vi "ExAdvPMAppCamera.vi"() -> ()   [LabVIEW 2010]
uses:
  Open-Close/CamHandle.vi
  GlobalCCDMaxDim.vi
  GlobalInitializeFlag.vi
  GlobalFramesToStr.vi
  GlobalTimingMode.vi
  GlobalAcquireFocusFlag.vi
  GlobalExposure.vi
  GlobalUserBin.vi
  GlobalBin2x.vi
  GlobalFullBin.vi
  GlobalFlipFlag.vi
  GlobalReverseFlag.vi
  GlobalIBackImgHndl.vi
  GlobalIFlatImgHndl.vi
panel:
  out "Camera Opened 2":bool
  out "Camera Opened":bool
  in  "Exit program":bool
  out "error out":errorcluster
  in  "error in (no error)":errorcluster
  in  "Tab Control":T1(tab)
  in  "Focus/Acquire Mode":u32=1 min=1 max=5 step=1
  in  "Number of Frames to store":u32=1 min=1 step=1
  in  "Intensifier":bool
  in  "Readout Port":i32=-1 min=-1 step=1
  in  "ADC Offset 2":i32=-1 min=-1 step=1
  in  "ADC Gain 2":i32=-1 min=-1 step=1
  in  "ADC speed":i32=-2 min=-3 step=1
  in  "Trigger Edge":u32(ring)=1 items=["N/A", "Positive (leading) edge", "Negative (falling) edge"]
  in  "Timing Mode":u32(ring)=1 items=["N/A", "Free Run/Timed", "Trigger First (PM only)", "Ext Sync/Strobed ", "Variable Exp (PM only)", "Flash Mode (PM only)"]
  out "Pixel Time":i32
  out "Bit Depth":i32
  out "ReadOut port":i32
  out "ADC Offset":i32
  out "ADC Gain":i32
  out "ADC Speed":i32
  in  "Set Experiment \nParameters, Initialize \nCamera/Controller":bool
  out "temperature":dbl format="%.2f"
  out "Temperature Read":dbl(slide) scale=-120.0..20.0
  in  "Temperature":dbl format="%.2f"
  in  "Exposure":dbl format="%.2f"
  out "Controller Initialized":bool
  out "Total":u32
  out "Y dim":u32
  out "X dim":u32
  in  "Y Bin":u32=1 min=1 step=1
  in  "Y End":u32=100 min=1 step=1
  in  "Y Start":u32=1 min=1 step=1
  in  "X Bin":u32=1 min=1 step=1
  in  "X End":u32=100 min=1 step=1
  in  "X Start":u32=1 min=1 step=1
  out "Bin 2":bool
  out "User":bool
  out "Full":bool
  in  "Binned by 2 Button":bool
  in  "User Defined Button":bool
  in  "Full CCD Button":bool
  out "Flip\nActive":bool
  in  "Flip flag Button":bool
  out "Reverse\nActive":bool
  in  "Image Reverse Button":bool
  out "Flat Field\nActive":bool
  out "Background \nActive":bool
  in  "Frame number to read":u32=1 min=1 step=1
  in  "Flat Button":bool
  in  "Back Button":bool
  in  "Full File Name":path
  in  "FileType":u32=67371008
  in  "SITKFULLDISPLAYLib.SITKFullDisplay":refnum<k7>(container)
  out "Reverse\nactive":bool
  out "Flip\nactive":bool
  out "Flat Field\nactive":bool
  out "background\nactive":bool
  in  "Reverse\nbutton":bool
  in  "Flip\nbutton":bool
  in  "Flat Field\nbutton":bool
  in  "Background\nbutton":bool
  in  "stop 2":bool
  in  "Start":bool
  out "Camera initialized":bool
  out "Collecting Data":bool
  in  "SITKFULLDISPLAYLib.SITKFullDisplay":refnum<k7>(container)
  in  "Full File Name\nfor Acqure":path
  in  "OK Button":bool
  out "camera initialized":bool
  # "Note: In order for any parameters to change and be downloaded the initialize button must be hit."
  # "The following are read \nfrom camera after setting\nvalues to left.\n-1 value means it isn't \nsupported by camera."
  # "For Slowest ADC speed set this to -3\nFor Fastest ADC speed set this to -2\nTo use current ADC speed don't  hook up or use -1\notherwise put speed in as kHz"
  # "To use current gain don't hook up or set to -1"
  # "To use current gain don't hook up or set to -1"
  # "To use current gain don't hook up or set to -1"
  # "Pixels coming back\nfrom Camera"
  # "NOTE: if background subtraction and/or flat field are being used and \nthe ROIs changed, there are no checks in this example for this."
  # "File Types:\nSPE = 67371008\nTIF   = 67174400\nPMI  = 67436544"
  # "Browse match pattern is set to *.spe.  Modify this if different file type is needed."
  # "Instructions:\nMake sure camera/controller has been initialized (LED should be on).\nPress start button, display should appear.\nWhen done press stop button, display should disappear.\nLive Operations buttons only work while collecting data, not before,\nto setup before goto On-Line operations tab."
  # "Live Operations, will only work while collecting data."
  # "Instructions:\nMake sure the camera/controller has been initialized.  The light should be on.\nMake sure to put in a file name with path to save data.\nPress Start button and display will pop up and data will be saved in file."
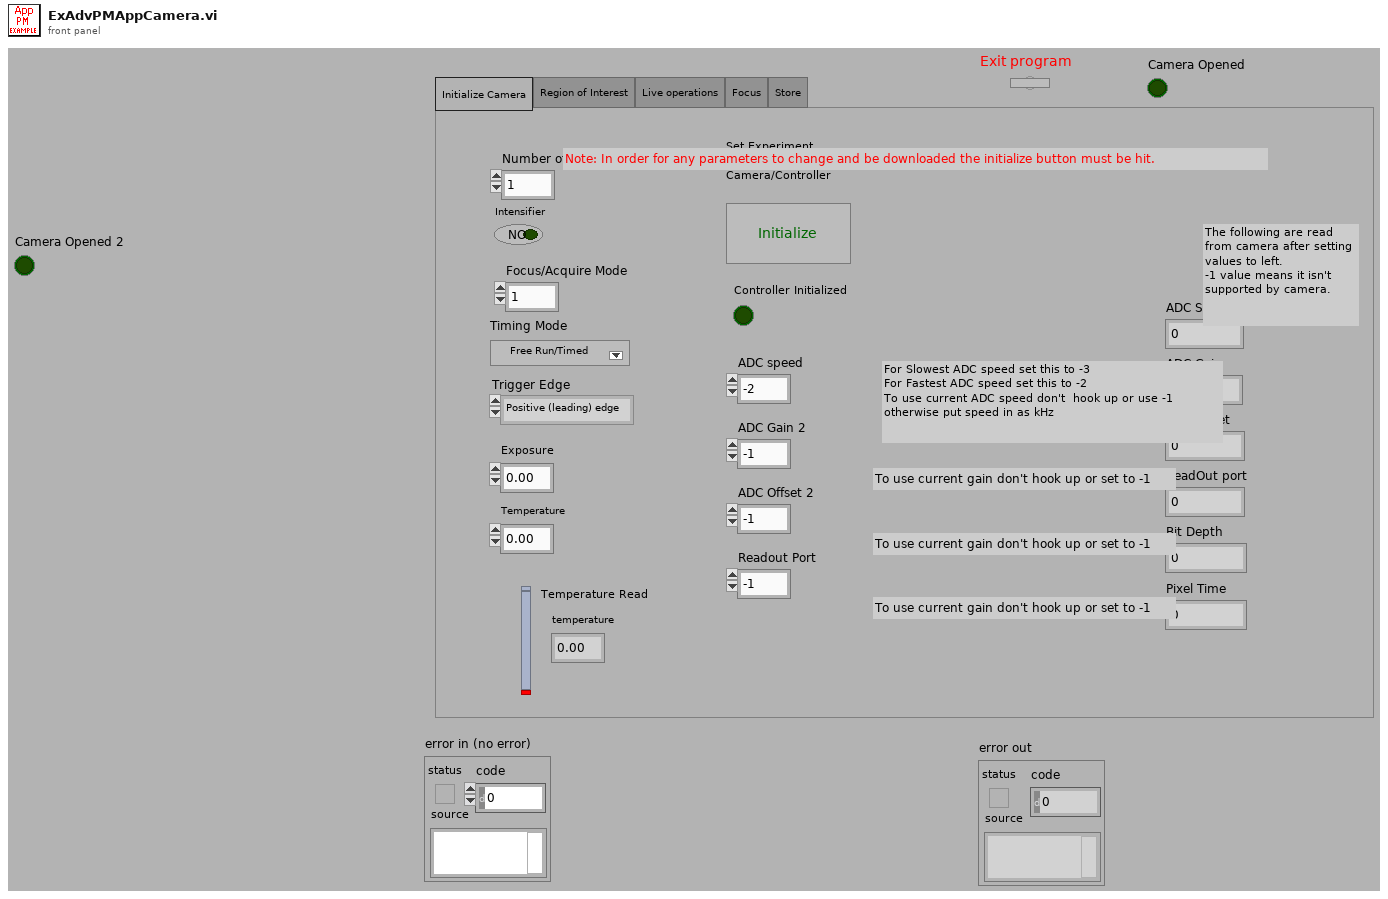
[diagram p1: front panel]
types:
  T1 = enum32{"Initialize Camera", "Region of Interest", "Live operations", "Focus", "Store"}
  T2 = cluster{"X Start":u32, "X End":u32, "X Bin":u32, "Y Start":u32, "Y End":u32, "Y Bin":u32}
  T3 = cluster{i32, "CCD Max X":u32, i32, i32, "CCD Max Y":u32, i32}
  T4 = cluster{"Camera Handle":u32, "Pulser Handle":u32, "File Handle":u32, "Display Handle":u32, "Image Handle":u32}
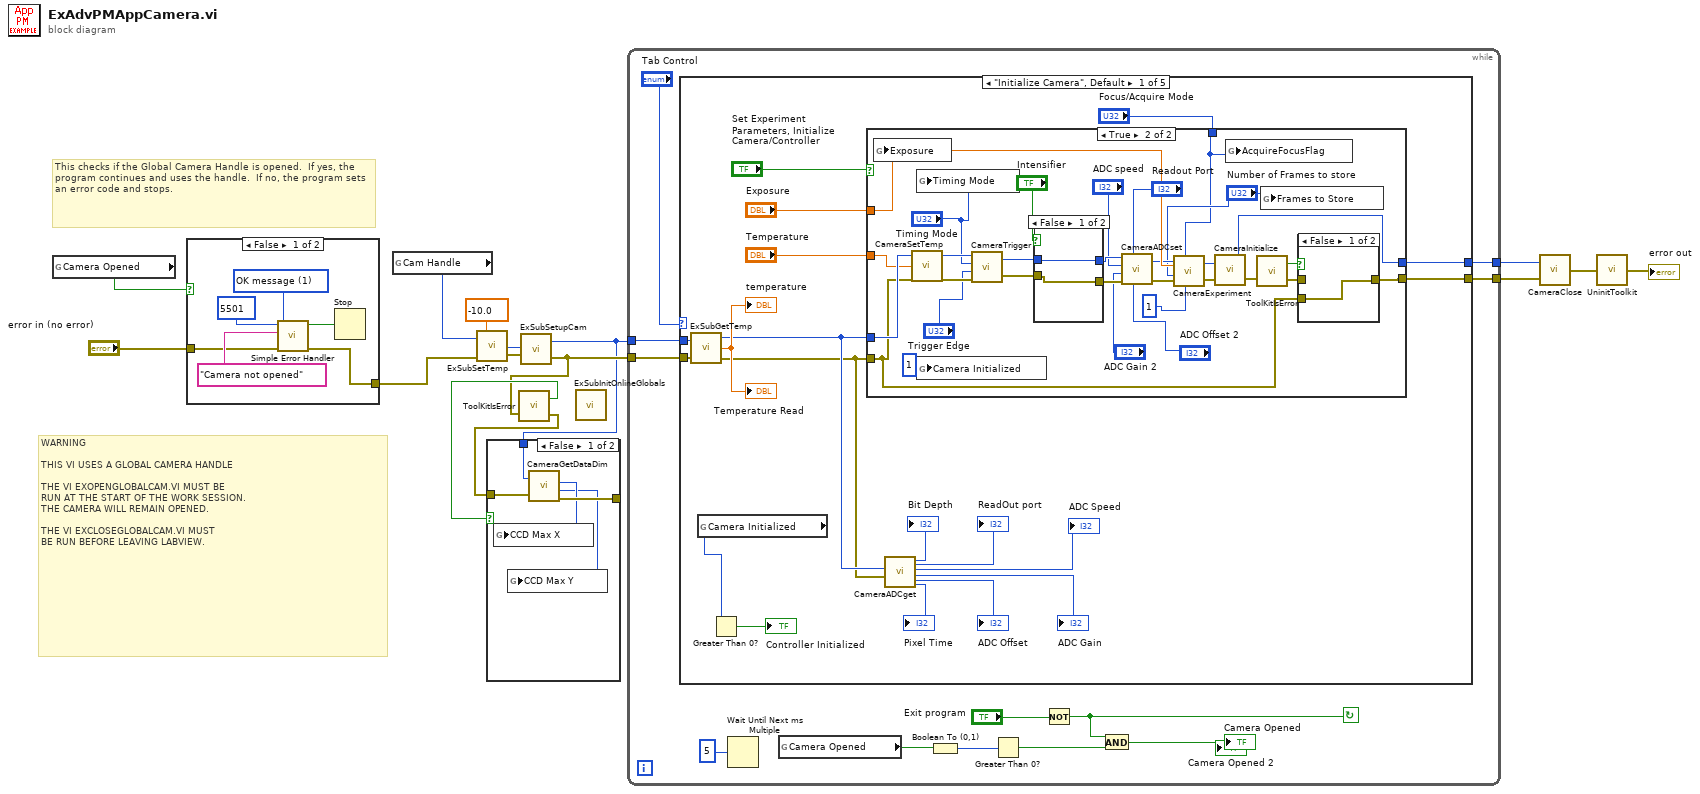
[diagram p0: block diagram]
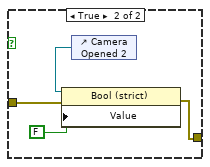
[diagram p2: hidden frame]
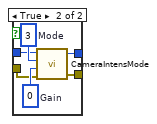
[diagram p6: hidden frame]
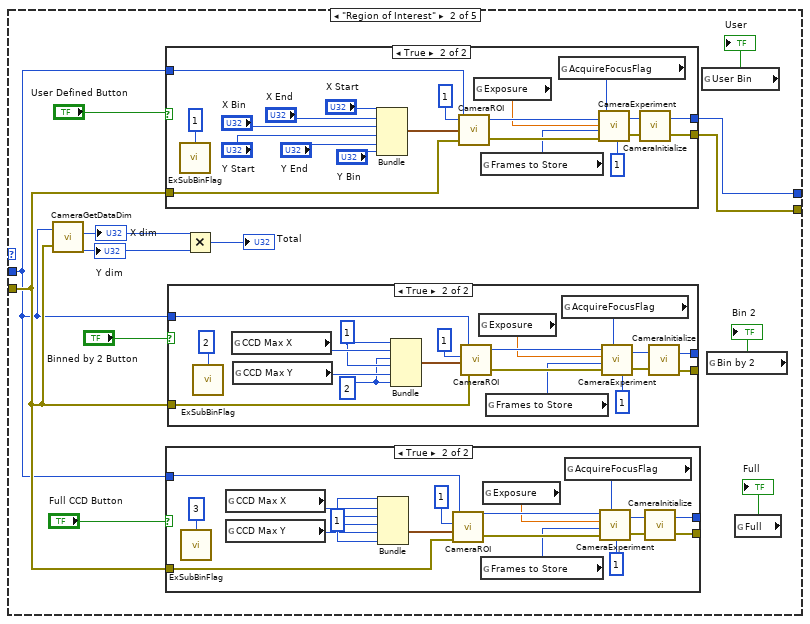
[diagram p7: hidden frame]
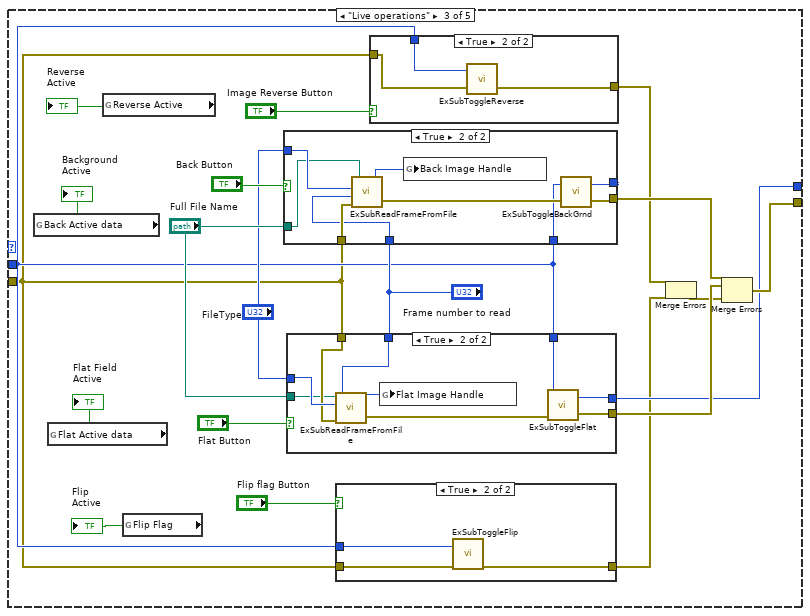
[diagram p11: hidden frame]
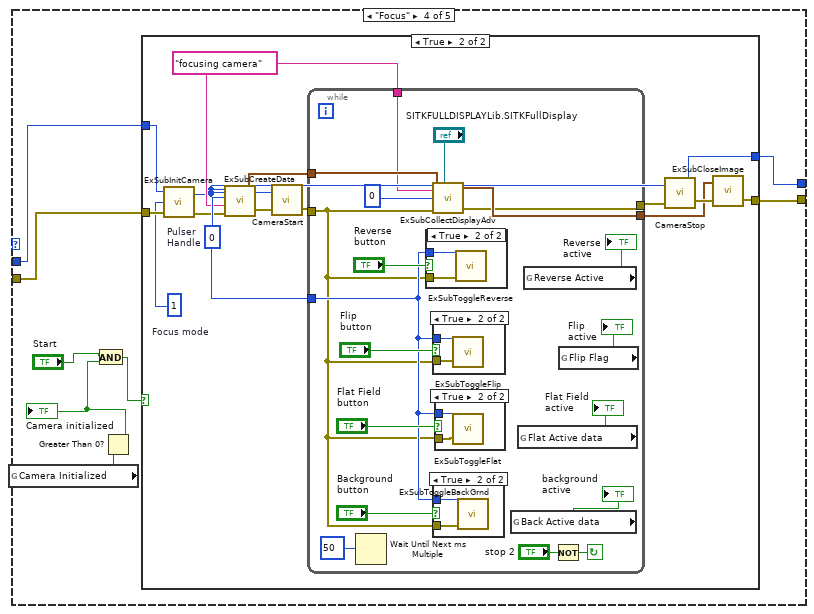
[diagram p16: hidden frame]
diagram:
  # "WARNING\n\nTHIS VI USES A GLOBAL CAMERA HANDLE\n\nTHE VI EXOPENGLOBALCAM.VI MUST BE\nRUN AT THE START OF THE WORK SESSION.\nTHE CAMERA WILL REMAIN OPENED.\n\nTHE VI EXCLOSEGLOBALCAM.VI MUST\nBE RUN BEFORE LEAVING LABVIEW."
  # "This checks if the Global Camera Handle is opened.  If yes, the program continues and uses the handle.  If no, the program sets\nan error code and stops."
  n1 = global read "CamHandle.vi" "Camera Opened"() -> (w4:bool)
  n2 = case shown="False" w4 {
    tunnel: "error in (no error)" -> [w17 w23]
    tunnel: [w16 w22] -> w2
    frame False {
      w21 = u16 1 items=["no dialog", "OK message", "continue or stop message"] ("type of dialog (OK msg:1)")
      n3 = call <vilib>:"Simple Error Handler.vi"("error code (no error:0)"=5501, "error source (\" \")"="Camera not opened", "type of dialog (OK msg:1)"=w21, "error in (no error)"=w17) -> ("error?"=w19:bool, "error out"=w16:errorcluster)  [unwired: 1 in, 3 out]
      n4 = Stop(stop? (T)=w19) -> ()
    }
    frame True {
      n5 = control-ref of="Camera Opened 2"() -> (w24:refnum<vi>)
      n6 = property class="Bool (strict)"(reference=w24, error in=w23, "Value"=FALSE) -> (error out=w22:errorcluster)  [unwired: 1 out]
    }
  }
  n7 = global read "CamHandle.vi" "Cam Handle"() -> (w1:u32)
  n8 = call "ExSubSetTemp.vi"("error in (no error)"=w2, "Temperature"=-10.0, "CameraHandle"=w1) -> ("error out"=w14:errorcluster, "Camera Handle"=w6:u32)
  n9 = call "ExSubSetupCam.vi"("error in (no error)"=w14, "Camera Handle"=w6) -> ("error out"=w7:errorcluster, "Camera Handle"=w5:u32)
  n10 = call <userlib>:"ToolKitIsError.vi"("error in"=w7) -> ("error out"=w8:errorcluster, "Error Flag"=w9:bool)  [unwired: 1 in]
  n11 = case shown="False" w9 {
    tunnel: w8 -> [w29 w31]
    tunnel: [w30 w31] -> _
    tunnel: w5 -> [w26 _]
    frame False {
      n12 = call <userlib>:"CameraGetDataDim.vi"("Camera Handle"=w26, "error in"=w29) -> ("Xdim"=w28:u32, "Ydim"=w27:u32, "error out"=w30:errorcluster)  [unwired: 1 out]
      n13 = global write "GlobalCCDMaxDim.vi" "CCD Max X"(w28) -> ()
      n14 = global write "GlobalCCDMaxDim.vi" "CCD Max Y"(w27) -> ()
    }
    frame True {
    }
  }
  n15 = call "ExSubInitOnlineGlobals.vi"() -> ()  [unwired: 1 in]
  n16 = while {
    tunnel: w5 -> [w43]
    tunnel: w7 -> [w40]
    tunnel: [w39] -> w13
    tunnel: [w38] -> w12
    stop <- w37 continue-if-true
    n17 = case shown="\"Initialize Camera\", Default" "Tab Control" {
      tunnel: w43 -> [w62 w110 w186 w233 w288]
      tunnel: w40 -> [w54 w111 w185 w232 w287]
      tunnel: [w46 w109 w193 w235 w285] -> w39
      tunnel: [w45 w108 w194 w234 w286] -> w38
      frame "Initialize Camera", Default {
        n18 = call "ExSubGetTemp.vi"("Camera Handle"=w62, "error in (no error)"=w54) -> ("Camera Handle"=w53:u32, "Temperature Real"=→"temperature" →"Temperature Read":dbl, "error out"=w52:errorcluster)
        n19 = global read "GlobalInitializeFlag.vi" "Camera Initialized"() -> (w57:u32)
        n20 = Greater Than 0?(x=w57) -> (x > 0?=→"Controller Initialized":bool)
        n21 = case shown="True" "Set Experiment \nParameters, Initialize \nCamera/Controller" {
          tunnel: "Exposure" -> [_ w83]
          tunnel: "Temperature" -> [_ w92]
          tunnel: w52 -> [w63 w67]
          tunnel: w53 -> [w64 w93]
          tunnel: [w63 w70] -> w45
          tunnel: [w64 w68] -> w46
          tunnel: "Focus/Acquire Mode" -> [_ w65]
          frame False {
          }
          frame True {
            n22 = global write "GlobalExposure.vi" "Exposure"(w83) -> ()
            n23 = call <userlib>:"CameraSetTemp.vi"("error in (no error)"=w67, "Temperature"=w92, "Camera Handle"=w93) -> ("error out"=w82:errorcluster, "Camera Handle"=w81:u32)
            n24 = global write "GlobalTimingMode.vi" "Timing Mode"("Timing Mode") -> ()
            n25 = global write "GlobalInitializeFlag.vi" "Camera Initialized"(1) -> ()
            n26 = call <userlib>:"CameraTrigger.vi"("error in"=w82, "Trigger Edge"="Trigger Edge", "Timing Mode"="Timing Mode", "Camera Handle"=w81) -> ("error out"=w78:errorcluster, "Camera Handle"=w79:u32)
            n27 = case shown="False" "Intensifier" {
              tunnel: [w98 w104] -> w89
              tunnel: [w97 w103] -> w90
              tunnel: w79 -> [w98 w100]
              tunnel: w78 -> [w97 w99]
              frame False {
              }
              frame True {
                w101 = u32 0  # Gain
                w102 = u32 3  # Mode
                n28 = call <userlib>:"CameraIntensMode.vi"("error in"=w99, "Intensifier Gain"=w101, "Mode"=w102, "Camera Handle"=w100) -> ("error out"=w103:errorcluster, "Camera Handle"=w104:u32)
              }
            }
            n29 = call <userlib>:"CameraADCset.vi"("ADC offset"="ADC Offset 2", "Read Out port"="Readout Port", "error in (no error)"=w90, "ADC Gain"="ADC Gain 2", "ADC Speed"="ADC speed", "Camera Handle"=w89) -> ("error out"=w76:errorcluster, "Camera Handle"=w75:u32)
            n30 = call <userlib>:"CameraExperiment.vi"("Number of Accumulations"=1, "Acquire / Focus Flag"=w65, "error in"=w76, "Number of Images"="Number of Frames to store", "Exposure (sec)"=w83, "Camera Handle"=w75) -> ("error out"=w74:errorcluster, "Camera Handle"=w73:u32)
            n31 = call <userlib>:"CameraInitialize.vi"("error in"=w74, "Camera Handle"=w73) -> ("error out"=w69:errorcluster, "Camera Handle"=w68:u32)
            n32 = global write "GlobalAcquireFocusFlag.vi" "AcquireFocusFlag"(w65) -> ()
            n33 = call <userlib>:"ToolKitIsError.vi"("error in"=w69) -> ("error out"=w71:errorcluster, "Error Flag"=w72:bool)  [unwired: 1 in]
            n34 = global write "GlobalFramesToStr.vi" "Frames to Store"("Number of Frames to store") -> ()
            n35 = case shown="False" w72 {
              tunnel: w71 -> [_ w96]
              tunnel: [w95 w96] -> w70
              tunnel: w67 -> [w95 _]
              frame False {
              }
              frame True {
              }
            }
          }
        }
        n36 = call <userlib>:"CameraADCget.vi"("Camera handle"=w53, "error in (no error)"=w52) -> ("Bit Depth"=→"Bit Depth":i32, "Pixel Time"=→"Pixel Time":i32, "Readout Port"=→"ReadOut port":i32, "ADC Offset"=→"ADC Offset":i32, "ADC Speed"=→"ADC Speed":i32, "ADC Gain"=→"ADC Gain":i32)  [unwired: 2 out]
      }
      frame "Region of Interest" {
        n37 = call <userlib>:"CameraGetDataDim.vi"("Camera Handle"=w110, "error in"=w111) -> ("Xdim"=w107:u32, "Ydim"=w106:u32)  [unwired: 2 out]
        "X dim" <- w107
        "Y dim" <- w106
        n38 = case shown="True" "User Defined Button" {
          tunnel: w110 -> [w160 w164]
          tunnel: [w160 w179] -> w109
          tunnel: w111 -> [w159 w163]
          tunnel: [w159 w176] -> w108
          frame False {
          }
          frame True {
            n39 = call "ExSubBinFlag.vi"("Binning \nUser = 1\nBin 2 = 2\nFull = 3"=1) -> ()
            n40 = Bundle("X Start"="X Start", "X End"="X End", "X Bin"="X Bin", "Y Start"="Y Start", "Y End"="Y End", "Y Bin"="Y Bin") -> (w165:T2)  [unwired: 1 in]
            n41 = call <userlib>:"CameraROI.vi"("error in"=w163, "ROI Params"=w165, "ROI Index"=1, "Camera Handle"=w164) -> ("error out"=w178:errorcluster, "Camera Handle"=w181:u32)
            n42 = global read "GlobalExposure.vi" "Exposure"() -> (w174:dbl)
            n43 = global read "GlobalFramesToStr.vi" "Frames to Store"() -> (w173:u32)
            n44 = global read "GlobalAcquireFocusFlag.vi" "AcquireFocusFlag"() -> (w172:u32)
            n45 = call <userlib>:"CameraExperiment.vi"("Number of Accumulations"=1, "Acquire / Focus Flag"=w172, "error in"=w178, "Number of Images"=w173, "Exposure (sec)"=w174, "Camera Handle"=w181) -> ("error out"=w177:errorcluster, "Camera Handle"=w180:u32)
            n46 = call <userlib>:"CameraInitialize.vi"("error in"=w177, "Camera Handle"=w180) -> ("error out"=w176:errorcluster, "Camera Handle"=w179:u32)
          }
        }
        n47 = case shown="True" "Full CCD Button" {
          tunnel: w110 -> [w119 w122]
          tunnel: [w119 w129] -> _
          tunnel: w111 -> [w118 w121]
          tunnel: [w118 w128] -> _
          frame False {
          }
          frame True {
            w127 = 1
            n48 = call "ExSubBinFlag.vi"("Binning \nUser = 1\nBin 2 = 2\nFull = 3"=3) -> ()
            n49 = global read "GlobalCCDMaxDim.vi" "CCD Max X"() -> (w126:u32)
            n50 = global read "GlobalCCDMaxDim.vi" "CCD Max Y"() -> (w125:u32)
            n51 = Bundle(w127, "CCD Max X"=w126, w127, w127, "CCD Max Y"=w125, w127) -> (w124:T3)  [unwired: 1 in]
            n52 = call <userlib>:"CameraROI.vi"("error in"=w121, "ROI Params"=w124, "ROI Index"=1, "Camera Handle"=w122) -> ("error out"=w135:errorcluster, "Camera Handle"=w137:u32)
            n53 = global read "GlobalFramesToStr.vi" "Frames to Store"() -> (w131:u32)
            n54 = global read "GlobalExposure.vi" "Exposure"() -> (w132:dbl)
            n55 = global read "GlobalAcquireFocusFlag.vi" "AcquireFocusFlag"() -> (w130:u32)
            n56 = call <userlib>:"CameraExperiment.vi"("Number of Accumulations"=1, "Acquire / Focus Flag"=w130, "error in"=w135, "Number of Images"=w131, "Exposure (sec)"=w132, "Camera Handle"=w137) -> ("error out"=w134:errorcluster, "Camera Handle"=w136:u32)
            n57 = call <userlib>:"CameraInitialize.vi"("error in"=w134, "Camera Handle"=w136) -> ("error out"=w128:errorcluster, "Camera Handle"=w129:u32)
          }
        }
        n58 = case shown="True" "Binned by 2 Button" {
          tunnel: w110 -> [w139 w144]
          tunnel: [w139 w150] -> _
          tunnel: w111 -> [w138 w145]
          tunnel: [w138 w149] -> _
          frame False {
          }
          frame True {
            w141 = 2
            w142 = 1
            n59 = call "ExSubBinFlag.vi"("Binning \nUser = 1\nBin 2 = 2\nFull = 3"=2) -> ()
            n60 = global read "GlobalCCDMaxDim.vi" "CCD Max X"() -> (w148:u32)
            n61 = global read "GlobalCCDMaxDim.vi" "CCD Max Y"() -> (w147:u32)
            n62 = Bundle(w142, "CCD Max X"=w148, w141, w142, "CCD Max Y"=w147, w141) -> (w146:T3)  [unwired: 1 in]
            n63 = call <userlib>:"CameraROI.vi"("error in"=w145, "ROI Params"=w146, "ROI Index"=1, "Camera Handle"=w144) -> ("error out"=w156:errorcluster, "Camera Handle"=w158:u32)
            n64 = global read "GlobalExposure.vi" "Exposure"() -> (w153:dbl)
            n65 = global read "GlobalFramesToStr.vi" "Frames to Store"() -> (w152:u32)
            n66 = global read "GlobalAcquireFocusFlag.vi" "AcquireFocusFlag"() -> (w151:u32)
            n67 = call <userlib>:"CameraExperiment.vi"("Number of Accumulations"=1, "Acquire / Focus Flag"=w151, "error in"=w156, "Number of Images"=w152, "Exposure (sec)"=w153, "Camera Handle"=w158) -> ("error out"=w155:errorcluster, "Camera Handle"=w157:u32)
            n68 = call <userlib>:"CameraInitialize.vi"("error in"=w155, "Camera Handle"=w157) -> ("error out"=w149:errorcluster, "Camera Handle"=w150:u32)
          }
        }
        n69 = Multiply(x=w107, y=w106) -> (x*y=→"Total":u32)
        n70 = global read "GlobalUserBin.vi" "User Bin"() -> (→"User":bool)
        n71 = global read "GlobalBin2x.vi" "Bin by 2"() -> (→"Bin 2":bool)
        n72 = global read "GlobalFullBin.vi" "Full"() -> (→"Full":bool)
      }
      frame "Live operations" {
        n73 = global read "GlobalIBackImgHndl.vi" "Back Active data"() -> (→"Background \nActive":bool)
        n74 = global read "GlobalIFlatImgHndl.vi" "Flat Active data"() -> (→"Flat Field\nActive":bool)
        n75 = global read "GlobalReverseFlag.vi" "Reverse Active"() -> (→"Reverse\nActive":bool)
        n76 = global read "GlobalFlipFlag.vi" "Flip Flag"() -> (→"Flip\nActive":bool)
        n77 = case shown="True" "Back Button" {
          tunnel: "Full File Name" -> [_ w229]
          tunnel: "FileType" -> [_ w230]
          tunnel: w185 -> [w222 w231]
          tunnel: [w222 w225] -> w196
          tunnel: "Frame number to read" -> [_ w228]
          tunnel: w186 -> [w221 w224]
          tunnel: [w221 w223] -> _
          frame False {
          }
          frame True {
            n78 = call "ExSubReadFrameFromFile.vi"("error in (no error)"=w231, "Frame to extract"=w228, "File type"=w230, "path to file to open"=w229) -> ("error out"=w226:errorcluster, "Image Handle"=w227:u32)
            n79 = global write "GlobalIBackImgHndl.vi" "Back Image Handle"(w227) -> ()
            n80 = call "ExSubToggleBackGrnd.vi"("error in (no error)"=w226, "Camera Handle"=w224) -> ("error out"=w225:errorcluster, "Camera Handle"=w223:u32)
          }
        }
        n81 = case shown="True" "Flat Button" {
          tunnel: "Full File Name" -> [_ w217]
          tunnel: "FileType" -> [_ w220]
          tunnel: w185 -> [w211 w218]
          tunnel: [w211 w213] -> w195
          tunnel: "Frame number to read" -> [_ w219]
          tunnel: w186 -> [w210 w215]
          tunnel: [w210 w214] -> w193
          frame False {
          }
          frame True {
            n82 = call "ExSubReadFrameFromFile.vi"("error in (no error)"=w218, "Frame to extract"=w219, "File type"=w220, "path to file to open"=w217) -> ("error out"=w212:errorcluster, "Image Handle"=w216:u32)
            n83 = global write "GlobalIFlatImgHndl.vi" "Flat Image Handle"(w216) -> ()
            n84 = call "ExSubToggleFlat.vi"("error in (no error)"=w212, "Camera Handle"=w215) -> ("error out"=w213:errorcluster, "Camera Handle"=w214:u32)
          }
        }
        n85 = case shown="True" "Flip flag Button" {
          tunnel: w186 -> [_ w209]
          tunnel: w185 -> [w206 w208]
          tunnel: [w206 w207] -> w184
          frame False {
          }
          frame True {
            n86 = call "ExSubToggleFlip.vi"("error in (no error)"=w208, "Camera Handle"=w209) -> ("error out"=w207:errorcluster)  [unwired: 1 out]
          }
        }
        n87 = case shown="True" "Image Reverse Button" {
          tunnel: w186 -> [_ w204]
          tunnel: w185 -> [w202 w205]
          tunnel: [w202 w203] -> w183
          frame False {
          }
          frame True {
            n88 = call "ExSubToggleReverse.vi"("error in (no error)"=w205, "Camera Handle"=w204) -> ("error out"=w203:errorcluster)  [unwired: 1 out]
          }
        }
        n89 = Merge Errors(w183, w184) -> (w182:errorcluster)
        n90 = Merge Errors(w196, w195, w182) -> (w194:errorcluster)
      }
      frame "Focus" {
        n91 = global read "GlobalInitializeFlag.vi" "Camera Initialized"() -> (w237:u32)
        n92 = Greater Than 0?(x=w237) -> (x > 0?=w236:bool)
        "Camera initialized" <- w236
        n93 = And(x="Start", y=w236) -> (x .and. y?=w239:bool)
        n94 = case shown="True" w239 {
          tunnel: w232 -> [w240 w246]
          tunnel: w233 -> [w241 w244]
          tunnel: [w241 w250] -> w235
          tunnel: [w240 w249] -> w234
          frame False {
          }
          frame True {
            w242 = 1  # Focus mode
            w247 = "focusing camera"
            w253 = u32 0  # Pulser  Handle
            n95 = call "ExSubInitCamera.vi"("error in (no error)"=w246, "Focus / Acquire Mode"=w242, "Camera Handle"=w244) -> ("error out"=w245:errorcluster, "Camera Handle"=w243:u32)
            n96 = call "ExSubCreateData.vi"("error in (no error)"=w245, "File and Display Name"=w247, "Pulser Handle"=w253, "Camera Handle"=w243) -> ("error out"=w254:errorcluster, "Handles Out"=w256:T4)
            n97 = call <userlib>:"CameraStart.vi"("error in"=w254, "Camera Handle"=w243) -> ("error out"=w255:errorcluster)  [unwired: 1 out]
            n98 = while {
              tunnel: w256 -> [w274]
              tunnel: w255 -> [w262]
              tunnel: [w272] -> w252
              tunnel: [w273] -> w248
              tunnel: w247 -> [w268]
              tunnel: w243 -> [w263]
              stop <- w270 continue-if-true
              n99 = Wait Until Next ms Multiple(millisecond multiple=u32 50) -> ()  [unwired: 1 out]
              n100 = case shown="True" "Reverse\nbutton" {
                tunnel: w262 -> [_ w283]
                tunnel: w263 -> [_ w282]
                frame False {
                }
                frame True {
                  n101 = call "ExSubToggleReverse.vi"("error in (no error)"=w283, "Camera Handle"=w282) -> ()  [unwired: 2 out]
                }
              }
              n102 = call "ExSubCollectDisplayAdv.vi"("Handle Cluster"=w274, "Display Title"=w268, "Store flag"=0, "error in (no error)"=w262, "advanced display handle"="SITKFULLDISPLAYLib.SITKFullDisplay") -> ("Handle Cluster Out"=w273:T4, "error out"=w272:errorcluster)  [unwired: 1 out]
              n103 = case shown="True" "Flip\nbutton" {
                tunnel: w263 -> [_ w280]
                tunnel: w262 -> [_ w281]
                frame False {
                }
                frame True {
                  n104 = call "ExSubToggleFlip.vi"("error in (no error)"=w281, "Camera Handle"=w280) -> ()  [unwired: 2 out]
                }
              }
              n105 = case shown="True" "Background\nbutton" {
                tunnel: w263 -> [_ w277]
                tunnel: w262 -> [_ w276]
                frame False {
                }
                frame True {
                  n106 = call "ExSubToggleBackGrnd.vi"("error in (no error)"=w276, "Camera Handle"=w277) -> ()  [unwired: 2 out]
                }
              }
              n107 = case shown="True" "Flat Field\nbutton" {
                tunnel: w263 -> [_ w278]
                tunnel: w262 -> [_ w279]
                frame False {
                }
                frame True {
                  n108 = call "ExSubToggleFlat.vi"("error in (no error)"=w279, "Camera Handle"=w278) -> ()  [unwired: 2 out]
                }
              }
              n109 = global read "GlobalIBackImgHndl.vi" "Back Active data"() -> (→"background\nactive":bool)
              n110 = global read "GlobalIFlatImgHndl.vi" "Flat Active data"() -> (→"Flat Field\nactive":bool)
              n111 = global read "GlobalReverseFlag.vi" "Reverse Active"() -> (→"Reverse\nactive":bool)
              n112 = Not(x="stop 2") -> (.not. x?=w270:bool)
              n113 = global read "GlobalFlipFlag.vi" "Flip Flag"() -> (→"Flip\nactive":bool)
            }
            n114 = call <userlib>:"CameraStop.vi"("error in"=w252, "Camera Handle"=w243) -> ("error out"=w251:errorcluster, "Camera Handle"=w250:u32)
            n115 = call "ExSubCloseImage.vi"("error in (no error)"=w251, "Handles In"=w248) -> ("error out"=w249:errorcluster)
          }
        }
      }
      frame "Store" {
        n116 = global read "GlobalInitializeFlag.vi" "Camera Initialized"() -> (w290:u32)
        n117 = Greater Than 0?(x=w290) -> (x > 0?=w289:bool)
        "camera initialized" <- w289
        n118 = And(x="OK Button", y=w289) -> (x .and. y?=w292:bool)
        n119 = case shown="True" w292 {
          tunnel: w288 -> [w294 w301]
          tunnel: w287 -> [w293 w296]
          tunnel: [w293 w304] -> w286
          tunnel: [w294 w299] -> w285
          frame False {
          }
          frame True {
            w298 = 2  # Store mode
            w313 = u32 0  # Pulser Handle
            n120 = property on="Collecting Data" class="Bool (strict)"(error in=w296, "Value"=TRUE) -> (error out=w295:errorcluster)  [unwired: 1 in, 1 out]
            n121 = Path To String(path="Full File Name\nfor Acqure") -> (string=w311:string)
            n122 = call "ExSubInitCamera.vi"("error in (no error)"=w295, "Focus / Acquire Mode"=w298, "Camera Handle"=w301) -> ("error out"=w300:errorcluster, "Camera Handle"=w299:u32)
            n123 = call "ExSubCreateFile.vi"("error in (no error)"=w300, "File and Display Name"=w311, "Pulser Handle"=w313, "Camera Handle"=w299) -> ("error out"=w314:errorcluster, "Handles Out"=w307:T4)
            n124 = call <userlib>:"CameraStart.vi"("error in"=w314, "Camera Handle"=w299) -> ("error out"=w308:errorcluster, "Camera Handle"=w305:u32)
            n125 = global read "GlobalFramesToStr.vi" "Frames to Store"() -> (w306:u32)
            n126 = call "ExSubNframeAdv.vi"("error in (no error)"=w308, "Display handle"="SITKFULLDISPLAYLib.SITKFullDisplay", "Number of Images"=w306, "Handle Cluster"=w307) -> ("error out"=w302:errorcluster, "Handle Cluster"=w310:T4)
            n127 = call <userlib>:"CameraStop.vi"("error in"=w302, "Camera Handle"=w305) -> ("error out"=w309:errorcluster)  [unwired: 1 out]
            n128 = call "ExSubCloseFileImage.vi"("error in (no error)"=w309, "Handles In"=w310) -> ("error out"=w304:errorcluster)
          }
        }
        "Collecting Data" <- FALSE
      }
    }
    n129 = Wait Until Next ms Multiple(millisecond multiple=5) -> ()  [unwired: 1 out]
    n130 = global read "CamHandle.vi" "Camera Opened"() -> (w33:bool)
    n131 = Boolean To (0,1)(Boolean=w33) -> (0, 1=w32:i16)
    n132 = Greater Than 0?(x=w32) -> (x > 0?=w36:bool)
    n133 = Not(x="Exit program") -> (.not. x?=w37:bool)
    n134 = And(x=w37, y=w36) -> (x .and. y?=→"Camera Opened":bool)
  }
  n135 = call <userlib>:"CameraClose.vi"("error in"=w12, "Camera Handle"=w13) -> ("error out"=w11:errorcluster)
  n136 = call <userlib>:"UninitToolkit.vi"("error in"=w11) -> ("error out"=→"error out":errorcluster)
